vi "power-test.vi"   [LabVIEW 2012, in "Mecanum Drive.lvrbt"]
uses:
  Mecanum Drive.lvrbt
  Serenity_mk2/SubVIs/auto_drive_TYP.ctl
types:
  T1 = typedef "auto_drive_TYP.ctl" = cluster{"Left X":i8, "Left Y":i8, "Right Y":i8, "Power (100)":i8, "Wait (ms)":u32, "Enc/Deg Target":i32, "Move Type":enum16{"Relative Degrees", "Wait", "Encoder"}}
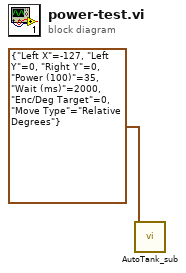
[diagram p0: block diagram]
diagram:
  n1 = call "AutoTank_sub.vi"("Drive Control"=T1 {"Left X"=-127, "Left Y"=0, "Right Y"=0, "Power (100)"=35, "Wait (ms)"=2000, "Enc/Deg Target"=0, "Move Type"=enum."Relative Degrees"}) -> ()  [unwired: 9 in, 2 out]
